vi "detectWC_v0.006.vi"(0 "gigaseal indiv":T1, 4 "breakin attempt #":i32, 5 "max breakin attempts #":i32, 9 "error in (no error)":errorcluster) -> (11 "error out":errorcluster, 14 "state out 2":T2=enum."Breaking in...")   [LabVIEW 2015]
uses:
  controls/user_message_v6.ctl
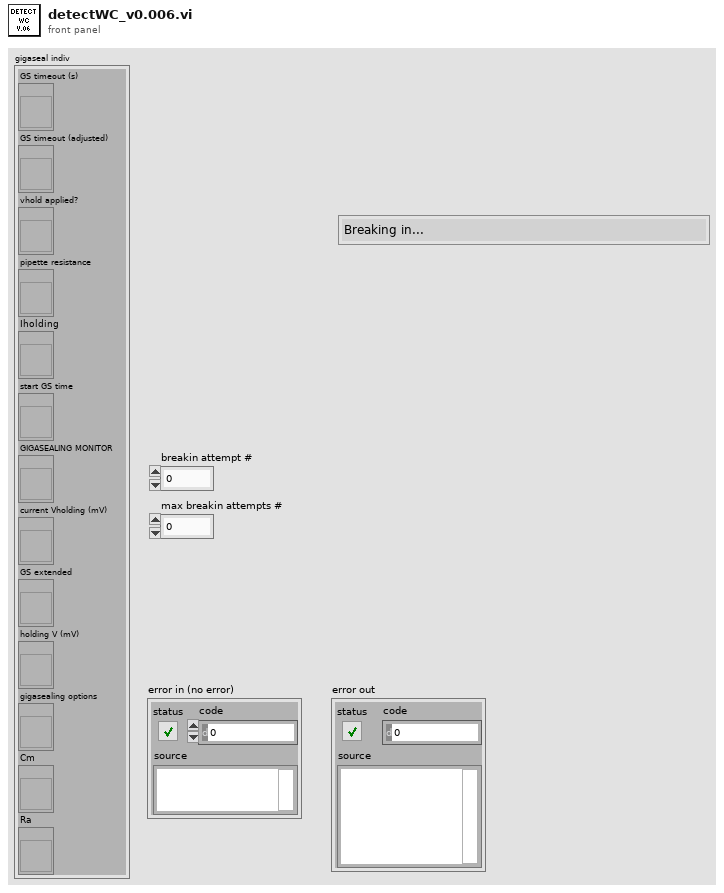
[diagram p1: front panel]
types:
  T1 = cluster{"GS timeout (s)":refnum<vi>, "GS timeout (adjusted)":refnum<vi>, "vhold applied?":refnum<vi>, "pipette resistance":refnum<vi>, "Iholding":refnum<vi>, "start GS time":refnum<vi>, "GIGASEALING MONITOR":refnum<vi>, "current Vholding (mV)":refnum<vi>, "GS extended":refnum<vi>, "holding V (mV)":refnum<vi>, "gigasealing options":refnum<vi>, "Cm":refnum<vi>, "Ra ":refnum<vi>}
  T2 = typedef "user_message_v6.ctl" = enum16{"Initializing...", "Setting defaults...", "Click OK to start patcherBot!", "Starting new attempt...", "Pipette repositioning...", "Initializing cell tracker...", "Gross approach...", "Human Positioning...", "In Process Calibration", "Detecting cell...", "Cell detected...", "Gigaseal Established...", "Breaking in...", "Successful breakin!", "Unsuccessful breakin!", "Whole-cell recording", "Saving autopatching parameters...", "Quitting VI", "Waiting for idle stage...", "Cleaning...", "Retracting pipette...", "DEBUG STATE", "Waiting to break in...", "Waiting for WC", "reclean", "Done with Current Set of Cells"}
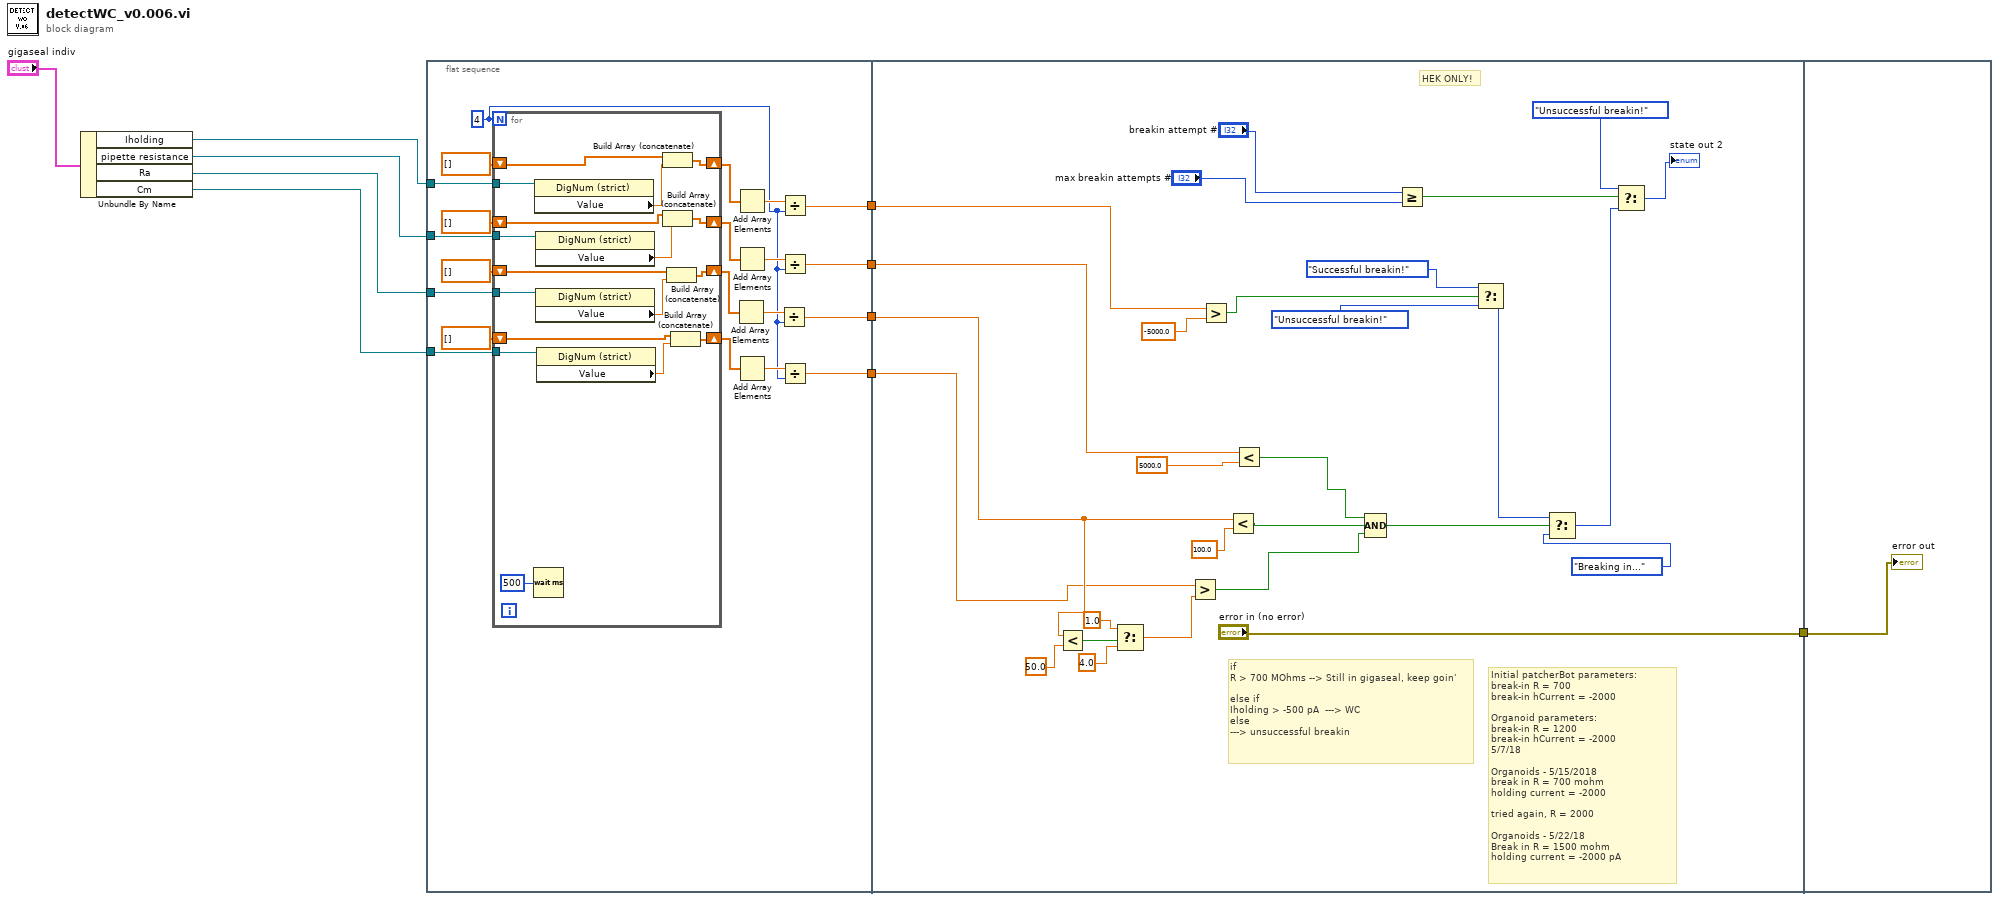
[diagram p0: block diagram]
diagram:
  n1 = Unbundle By Name("gigaseal indiv") -> ("Iholding"=w8:refnum<vi>, "pipette resistance"=w7:refnum<vi>, "Ra"=w6:refnum<vi>, "Cm"=w5:refnum<vi>)
  n2 = flat-sequence {
    tunnel: w8 -> [w31]
    tunnel: w7 -> [w30]
    tunnel: w6 -> [w29]
    tunnel: w5 -> [w28]
    tunnel: [w14] -> w4
    tunnel: [w13] -> w3
    tunnel: [w12] -> w2
    tunnel: [w11] -> w1
    tunnel: ["error in (no error)"] -> w10
    tunnel: w4 -> [w52]
    tunnel: w3 -> [w51]
    tunnel: w2 -> [w50]
    tunnel: w1 -> [w49]
    tunnel: w10 -> [w77]
    frame #0 {
      w19 = 4
      n3 = for {
        N: w19 -> [_]
        tunnel: w31 -> [w47]
        tunnel: w30 -> [w46]
        tunnel: w29 -> [w45]
        tunnel: w28 -> [w44]
        shift-right: [w42] -> w27
        shift-left: dbl[] [] -> [w38]
        shift-right: [w40] -> w22
        shift-left: dbl[] [] -> [w39]
        shift-right: [w36] -> w21
        shift-left: dbl[] [] -> [w35]
        shift-right: [w33] -> w20
        shift-left: dbl[] [] -> [w32]
        n4 = Wait (ms)(milliseconds to wait=u32 500) -> ()  [unwired: 1 out]
        n5 = property class="DigNum (strict)"(reference=w47) -> ("Value"=w43:dbl)  [unwired: 1 in, 2 out]
        n6 = property class="DigNum (strict)"(reference=w46) -> ("Value"=w41:dbl)  [unwired: 1 in, 2 out]
        n7 = property class="DigNum (strict)"(reference=w45) -> ("Value"=w37:dbl)  [unwired: 1 in, 2 out]
        n8 = property class="DigNum (strict)"(reference=w44) -> ("Value"=w34:dbl)  [unwired: 1 in, 2 out]
        n9 = Build Array (concatenate)(w38, w43) -> (w42:dbl[])
        n10 = Build Array (concatenate)(w39, w41) -> (w40:dbl[])
        n11 = Build Array (concatenate)(w35, w37) -> (w36:dbl[])
        n12 = Build Array (concatenate)(w32, w34) -> (w33:dbl[])
      }
      n13 = Add Array Elements(numeric array=w21) -> (sum=w24:dbl)
      n14 = Add Array Elements(numeric array=w27) -> (sum=w26:dbl)
      n15 = Add Array Elements(numeric array=w22) -> (sum=w25:dbl)
      n16 = Add Array Elements(numeric array=w20) -> (sum=w23:dbl)
      n17 = Divide(x=w24, y=w19) -> (x/y=w12:dbl)
      n18 = Divide(x=w26, y=w19) -> (x/y=w14:dbl)
      n19 = Divide(x=w25, y=w19) -> (x/y=w13:dbl)
      n20 = Divide(x=w23, y=w19) -> (x/y=w11:dbl)
    }
    frame #1 {
      # "Initial patcherBot parameters:\nbreak-in R = 700\nbreak-in hCurrent = -2000\n\nOrganoid parameters:\nbreak-in R = 1200\nbreak-in hCurrent = -2000\n5/7/18\n\nOrganoids - 5/15/2018\nbreak in R = 700 mohm\nholding current = -2000\n\ntried again, R = 2000\n\nOrganoids - 5/22/18\nBreak in R = 1500 mohm\nholding current = -2000 pA"
      # "HEK ONLY!"
      # "if \nR > 700 MOhms --> Still in gigaseal, keep goin'\n\nelse if\nIholding > -500 pA  ---> WC\nelse\n---> unsuccessful breakin"
      n21 = Less?(x=w50, y=50.0) -> (x < y?=w54:bool)
      n22 = Select(t=1.0 ("y"), s=w54, f=4.0) -> (s? t:f=w57:dbl)
      n23 = Greater?(x=w49, y=w57) -> (0:w62:bool)
      n24 = Greater?(x=w52, y=-5000.0) -> (0:w69:bool)
      n25 = Less?(x=w50, y=100.0) -> (x < y?=w63:bool)
      n26 = Less?(x=w51, y=5000.0) -> (x < y?=w64:bool)
      n27 = Compound Arithmetic op=AND(w64, w63, w62) -> (w61:bool)
      n28 = Greater Or Equal?(x="breakin attempt #", y="max breakin attempts #") -> (x >= y?=w70:bool)
      n29 = Select(t=user_message_v6."Successful breakin!" ("state out"), s=w69, f=user_message_v6."Unsuccessful breakin!" ("state out")) -> (s? t:f=w60:T2)
      n30 = Select(t=w60, s=w61, f=user_message_v6."Breaking in..." ("state out")) -> (s? t:f=w71:T2)
      n31 = Select(t=user_message_v6."Unsuccessful breakin!" ("state out"), s=w70, f=w71) -> (s? t:f=→"state out 2":T2)
    }
    frame #2 {
      "error out" <- w77
    }
  }
